vi "Read all txt files to numeric array.vi"(3 "error in (no error)":errorcluster, 4 "format string (%d)":string="%d", 5 "selected folder":path) -> (0 "error out":errorcluster, 1 "Max Array Size":i32, 2 "Data Out":i32[][](array[numeric]))   [LabVIEW 2012]
panel:
  out "execution time (ms)":u32
  out "file data":i32[](array[numeric])
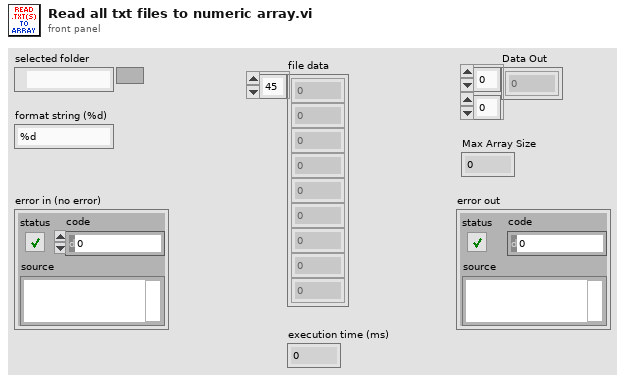
[diagram p1: front panel]
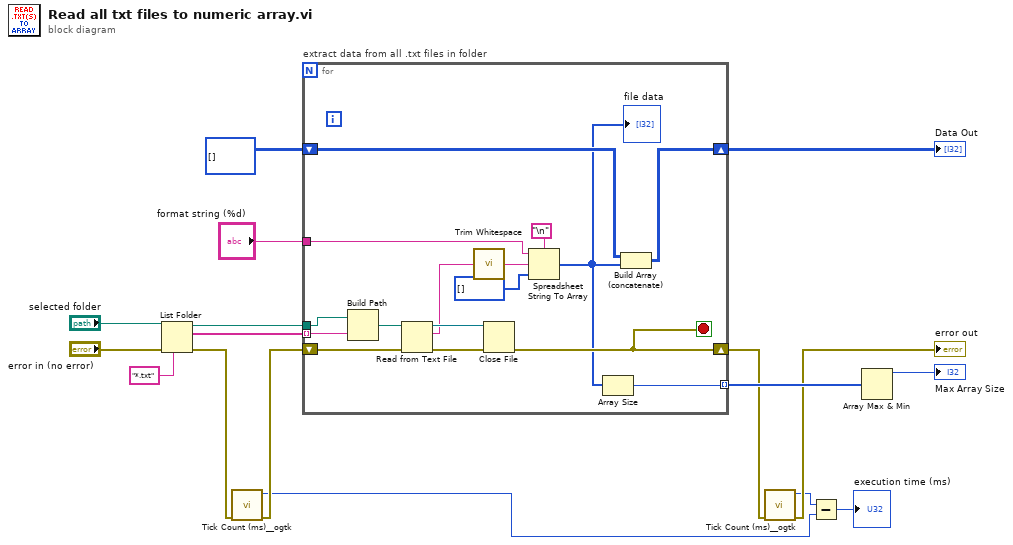
[diagram p0: block diagram]
diagram:
  n1 = List Folder(path="selected folder", pattern="*.txt", error in="error in (no error)") -> (path out=w10:path, filenames=w11:string[], error out=w7:errorcluster)  [unwired: 1 in, 1 out]
  n2 = call <userlib>:"Tick Count (ms)__ogtk.vi"("error in (no error)"=w7) -> ("error out"=w6:errorcluster, "millisecond timer value"=w2:u32)  [unwired: 9 in]
  n3 = for "extract data from all .txt files in folder" {
    shift-right: [w29] -> w5
    shift-left: w6 -> [w30]
    tunnel: w10 -> [w32]
    tunnel: w11 -> [w33] mode=indexing
    shift-right: [w28] -> w13
    shift-left: i32[][] [] -> [w27]
    tunnel: [w25] -> w9 mode=indexing
    tunnel: "format string (%d)" -> [w24]
    stop <- w29 stop-if-true
    n4 = Build Path(base path=w32, name or relative path=w33) -> (appended path=w31:path)
    n5 = Read from Text File(file (use dialog)=w31, error in=w30) -> (refnum out=w22:refnum<file>, text=w19:string, error out=w23:errorcluster)  [unwired: 2 in, 1 out]
    n6 = call <vilib>:"Trim Whitespace.vi"("string"=w19) -> ("trimmed string"=w18:string)  [unwired: 1 in]
    n7 = Close File(refnum=w22, error in=w23) -> (error out=w29:errorcluster)  [unwired: 1 out]
    n8 = Spreadsheet String To Array(delimiter (Tab)="\n", format string=w24, spreadsheet string=w18, array type (2D Dbl)=i32[] []) -> (array=w26:i32[])
    "file data" <- w26
    n9 = Array Size(array=w26) -> (size(s)=w25:i32)
    n10 = Build Array (concatenate)(w27, w26) -> (w28:i32[][])
  }
  "Data Out" <- w13
  n11 = call <userlib>:"Tick Count (ms)__ogtk.vi"("error in (no error)"=w5) -> ("error out"=→"error out":errorcluster, "millisecond timer value"=w3:u32)  [unwired: 9 in]
  n12 = Subtract(x=w3, y=w2) -> (x-y=→"execution time (ms)":u32)
  n13 = Array Max & Min(array=w9) -> (max value=→"Max Array Size":i32)  [unwired: 3 out]
